vi "Launch TCP Writers.vi"(8 "error in (no error)":errorcluster, 11 "Guardian in":refnum<class "Guardian.lvclass">) -> (0 "error out":errorcluster, 3 "Guardian out":refnum<class "Guardian.lvclass">)   [LabVIEW 2026, in "TALOS.lvlib" / "Guardian.lvlib" / "Guardian.lvclass"]
uses:
  Guardian.lvclass
  C:/LabVIEW Code/TALOS/builds/Actor Framework PPL/Actor Framework.lvlibp/1abvi3w/vi.lib/ActorFramework/Actor/Actor.lvclass
  C:/LabVIEW Code/TALOS/talos/Ancestor/Ancestor/Ancestor.lvclass
  Ancestor/Ancestor/Ancestor.lvclass/Ancestor.ctl
  Guardian.lvclass/Guardian.ctl
  Guardian Messages/Launch uService Msg/Launch uService Msg.lvclass/Launch uService Msg.ctl
  Ancestor/Ancestor/Read ID.vi
  Support VIs/Generate Error.vi
  FGV/Error Memory/Get Error Description.vi
  Support VIs/Get PC name.vi
  Support VIs/Get Class Name.vi
  <vilib>/Utility/error.llb/Clear Errors.vi
  FGV/Error Memory/Error Memory Core.vi
  <vilib>/AdvancedString/Delimited String to 1D String Array.vi
  <vilib>/AdvancedString/Delimited String to 1D String Array (string).vi
  Support VIs/Circus Root Path.vi
  FGV/Error Memory/Error Crt Lvl checker.vi
  FGV/Error Memory/Error Memory Core.vi/40c8088d-b597-4017-91af-faa98e00292e.vi
  FGV/Error Memory/Error Memory Core.vi/d4a3ab98-063c-4e44-b43d-fbdcfe6c2be2.vi
  Support VIs/Global Memory.vi
  <vilib>/Utility/LVClass/Get LV Class Name.vi
  Support VIs/Is in Packed Library.vi
  Support VIs/TALOS Root path.vi
  Support VIs/Read CSV worksheet.vi
  Support VIs/Global Constants.vi
  <vilib>/Utility/error.llb/General Error Handler.vi
  <vilib>/Utility/config.llb/Open Config Data.vi
  <vilib>/Utility/config.llb/Get Section Names.vi
  <vilib>/Utility/config.llb/Get Key Names.vi
  <vilib>/Utility/config.llb/Read Key.vi
  <vilib>/Utility/config.llb/Read Key (String).vi
  <vilib>/Utility/config.llb/Close Config Data.vi
  builds/Actor Framework PPL/Actor Framework.lvlibp/1abvi3w/vi.lib/ActorFramework/Message Enqueuer/Enqueue.vi
  Ancestor/Ancestor/Ancestor.lvclass
  <vilib>/Comparison/Equal/Equal Functor/Equal Functor.lvclass
  Guardian Messages/Launch uService Msg/Launch uService Msg.lvclass
  Classes/Guardian List/Guardian List.lvclass
  TALOS.lvlib
  builds/Actor Framework PPL/Actor Framework.lvlibp/1abvi3w/vi.lib/ActorFramework/Actor/Actor.lvclass
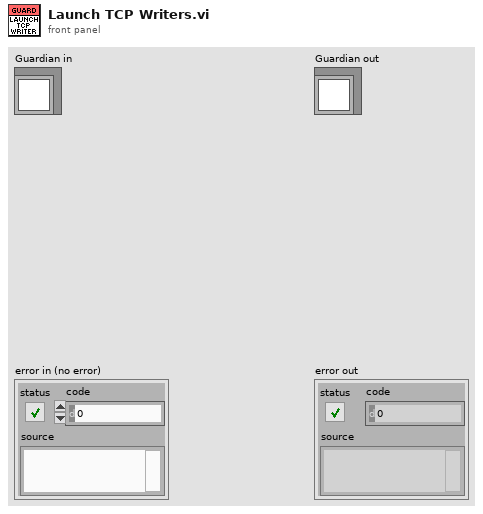
[diagram p1: front panel]
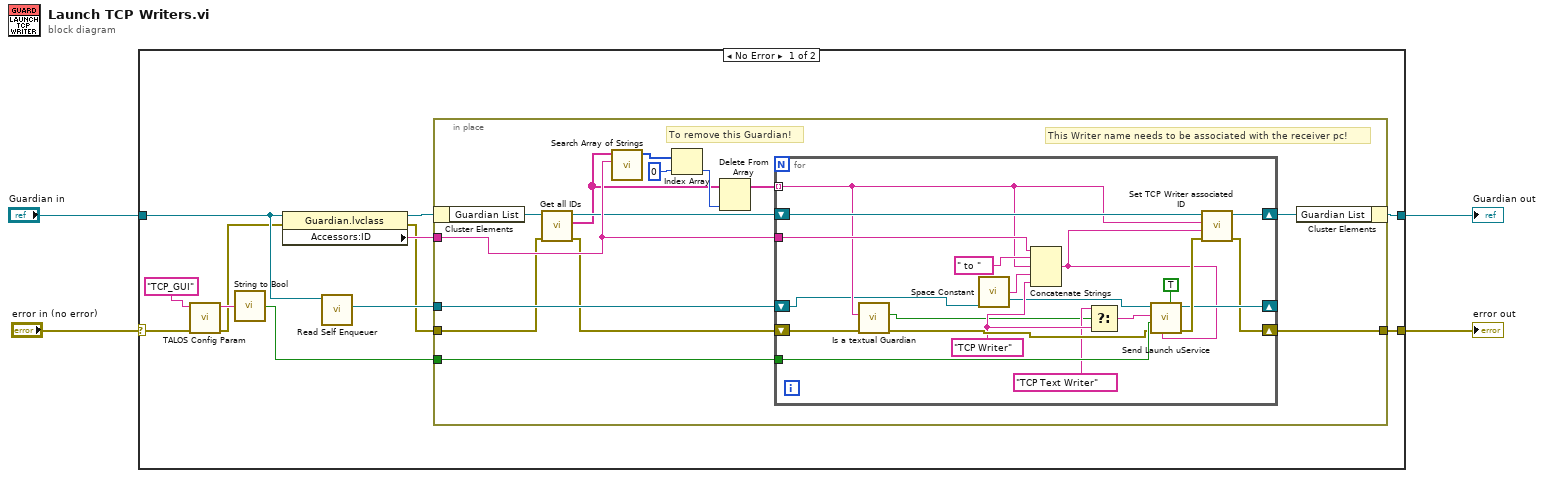
[diagram p0: block diagram]
diagram:
  n1 = case shown="No Error" "error in (no error)" {
    selector: "error in (no error)" -> [w7 w50]
    tunnel: [w16 w51] -> w4
    tunnel: [w15 w50] -> w3
    tunnel: "Guardian in" -> [w8 w51]
    frame No Error {
      n2 = call "TALOS Config Param.vi"("error in (no error)"=w7, "Parameter Name"="TCP_GUI") -> ("error out"=w6:errorcluster, "Output"=w12:string)  [unwired: 8 in]
      n3 = call "String to Bool.vi"("String"=w12) -> ("Boolean"=w11:bool)
      n4 = property class="Guardian.lvclass"(reference=w8, error in=w6) -> (reference out=w14:refnum<class "Guardian.lvclass">, error out=w5:errorcluster, "Accessors:ID"=w13:string)
      n5 = call "Read Self Enqueuer.vi"("Actor"=w8) -> ("Self Enqueuer"=w9:refnum<class "Message Enqueuer.lvclass">)  [unwired: 10 in]
      n6 = in-place {
        in-place-border: w9 -> [w30]
        in-place-border: [w29] -> w15
        in-place-border: w5 -> [w19]
        in-place-border: w13 -> [w24]
        in-place-border: w11 -> [w17]
        # "This Writer name needs to be associated with the receiver pc!"
        # "To remove this Guardian!"
        n7 = in-place-cluster #1(w14) -> ("Guardian List"=w22:refnum<class "Guardian List.lvclass">)
        n8 = call-dynamic "Get all IDs.vi"("error in (no error)"=w19, "Guardian List in"=w22) -> ("error out"=w18:errorcluster, "All IDs"=w20:string[], "Guardian List out"=w21:refnum<class "Guardian List.lvclass">)  [unwired: 7 in]
        n9 = call "Search Array of Strings.vi"("search string"=w24, "Search array"=w20) -> ("indices"=w27:i32[])  [unwired: 8 in, 1 out]
        n10 = Index Array(array=w27, index=0) -> (element=w28:i32)
        n11 = Delete From Array(array=w20, index=w28) -> (array with subset deleted=w25:string[])  [unwired: 1 in, 1 out]
        n12 = for {
          shift-right: [w41] -> w29
          shift-left: w18 -> [w39]
          tunnel: w25 -> [w33] mode=indexing
          shift-right: [w45] -> _
          shift-left: w30 -> [w32]
          tunnel: w24 -> [w37]
          shift-right: [w40] -> w23
          shift-left: w21 -> [w48]
          tunnel: w17 -> [w44]
          w35 = "TCP Writer" ("uService Class Name")
          n13 = call "Is a textual Guardian.vi"("error in (no error)"=w39, "Target GD ID"=w33) -> ("error out"=w38:errorcluster, "Textual?"=w31:bool)  [unwired: 8 in]
          n14 = call <vilib>:"Space Constant.vi"() -> ("String"=w46:string)
          n15 = Concatenate Strings(w37, " to " ("string"), w33, w46, w35) -> (w43:string)
          n16 = Select(t="TCP Text Writer" ("uService Class Name"), s=w31, f=w35) -> (s? t:f=w36:string)
          n17 = call "Send Launch uService.vi"("Highlander?"=TRUE, "uService ID"=w43, "error in (no error)"=w38, "GUI?"=w44, "uService Class Name"=w36, "Message Enqueuer"=w32) -> ("error out"=w47:errorcluster, "Message Enqueuer out"=w45:refnum<class "Message Enqueuer.lvclass">)  [unwired: 4 in]
          n18 = call-dynamic "Set TCP Writer associated ID.vi"("error in (no error)"=w47, "TCP Writer associated ID"=w43, "ID"=w33, "Guardian List in"=w48) -> ("error out"=w41:errorcluster, "Guardian List out"=w40:refnum<class "Guardian List.lvclass">)  [unwired: 6 in]
        }
        n19 = in-place-cluster #1("Guardian List"=w23) -> (w16:refnum<class "Guardian.lvclass">)
      }
    }
    frame Error {
    }
  }
  "Guardian out" <- w4
  "error out" <- w3
